vi "globalDevices.vi"() -> ()   [LabVIEW 2017]
panel:
  out "hamamatsuFrameReferences":refnum<data-value>[](array[refnum])
  out "ludlError":errorcluster
  in  "ludlPort":refnum<visa-resource-name>="COM1"
  out "daqVolumeFileError":errorcluster
  out "daqVolumeFileRefnum":refnum<file>
  in  "autofocusAidStage":u16(ring) items=["none", "focusKnob"]
  out "flashTask":refnum<k21>
  out "flashError":errorcluster
  in  "flashDigitalLine":tag="Dev1/port0/line2"
  in  "focusKnobSpeed":u8=255
  out "focusKnobError":errorcluster
  in  "focusKnobPort":refnum<visa-resource-name>="COM1"
  out "piezoUSBLastWrittenPos (um)":dbl
  out "piezoUSBError":i32
  out "piezoUSBHandle":i32
  out "csuShutterLastStatus":bool
  out "csuError":errorcluster
  in  "csuPort":refnum<visa-resource-name>="COM1"
  in  "galvoDY":dbl=0.08
  in  "galvoDX":dbl=0.08
  in  "galvoY0":dbl=0.05
  in  "galvoX0":dbl=-0.03
  out "hamamatsuSubtractBG":bool=TRUE
  out "daqFileError":errorcluster
  out "daqFileRefnum":refnum<file>
  in  "daqAOBufferSize":i32=8191
  in  "piezoReadVolTimingThresh":dbl
  out "piezoReadVolTimingError":errorcluster
  out "piezoReadVolTimingTask":refnum<k21>
  in  "piezoReadVolTimingChannel":tag="Dev1/ai1"
  in  "piezoWriteFunctionType":u16(ring) items=["triangle", "sine"]
  in  "galvoWriteMinVal":dbl=-10.0
  in  "galvoWriteMaxVal":dbl=10.0
  out "galvoYWriteError":errorcluster
  out "galvoXWriteError":errorcluster
  out "galvoYWriteTask":refnum<k21>
  out "galvoXWriteTask":refnum<k21>
  in  "galvoVoltsPerDegree":dbl=0.8
  in  "galvoYWriteChannel":tag="Dev2/ao0"
  in  "galvoXWriteChannel":tag="Dev2/ao1"
  in  "pharosClockRate":dbl=500000.0
  out "piezoWriteInitAtCenter":bool=TRUE
  out "piezoWriteInitRamp":dbl[](array[numeric])
  in  "piezoWriteSamplingRate":dbl=5000.0
  out "filterWheelInitialStatus":string
  out "filterWheelError":errorcluster
  in  "filterWheelPort":refnum<visa-resource-name>="COM1"
  in  "piezoWriteMaxVal":dbl=10.0
  out "hamamatsuStartTriggerMode":bool
  in  "piezoReadMinVal":dbl format="%0.2f"
  in  "piezoReadMaxVal":dbl=10.0 format="%0.2f"
  in  "piezoReadChannel":tag="Dev1/ai0"
  in  "hamamatsuFrameCounterTerminal":tag="/Dev1/PFI1"
  out "pharosError":errorcluster
  out "pharosTask":refnum<k21>
  in  "pharosDigitalLine":tag="Dev1/port0/line0"
  out "hamamatsuFrameCounterError":errorcluster
  out "hamamatsuFrameCounterTask":refnum<k21>
  in  "hamamatsuFrameCounterChannel":tag="Dev1/ctr0"
  in  "hamamatsuBufferSize":i32=200
  out "hamamatsuError":errorcluster {"code" format="%.0x"}
  out "hamamatsuBufferInfo":T1
  out "hamamatsuImageType":u32
  out "hamamatsuHandle":u32
  out "piezoWriteError":errorcluster
  out "piezoWriteTask":refnum<k21>
  in  "piezoWriteChannel":tag="Dev1/ao0"
  in  "piezo V/um":dbl=0.05
  out "piezoReadError":errorcluster
  out "piezoReadTask":refnum<k21>
  out "xboxError":errorcluster
  out "xboxID":refnum<k1>
  out "stageError":errorcluster
  out "stageIDs":cluster{"opaque pointer":u64, "id":i32}
  # "XBOX CONTROLLER"
  # "PIEZO"
  # "PHAROS"
  # "GALVO"
  # "STAGE (STANDA)"
  # "HAMAMATSU"
  # "FILTER WHEEL"
  # "Output (out from piezo)"
  # "Input (into piezo)"
  # "The galvo is mounted \"reversed\"\nwrt the labels on the motors. The\nmotor labelled \"X\" moves in Y and\nthe motor labelled \"Y\" moves in X.\n\nHere, I use the actual directions,\nnot the ones on the labels."
  # "CSU"
  # "FLASH"
  # "GENERAL DAQ"
  # "Volume timing"
  # "Frame counter"
  # "FOCUS KNOB"
  # "LUDL STAGE"
  # "USB connection"
  # "HARDWR CONFIG."
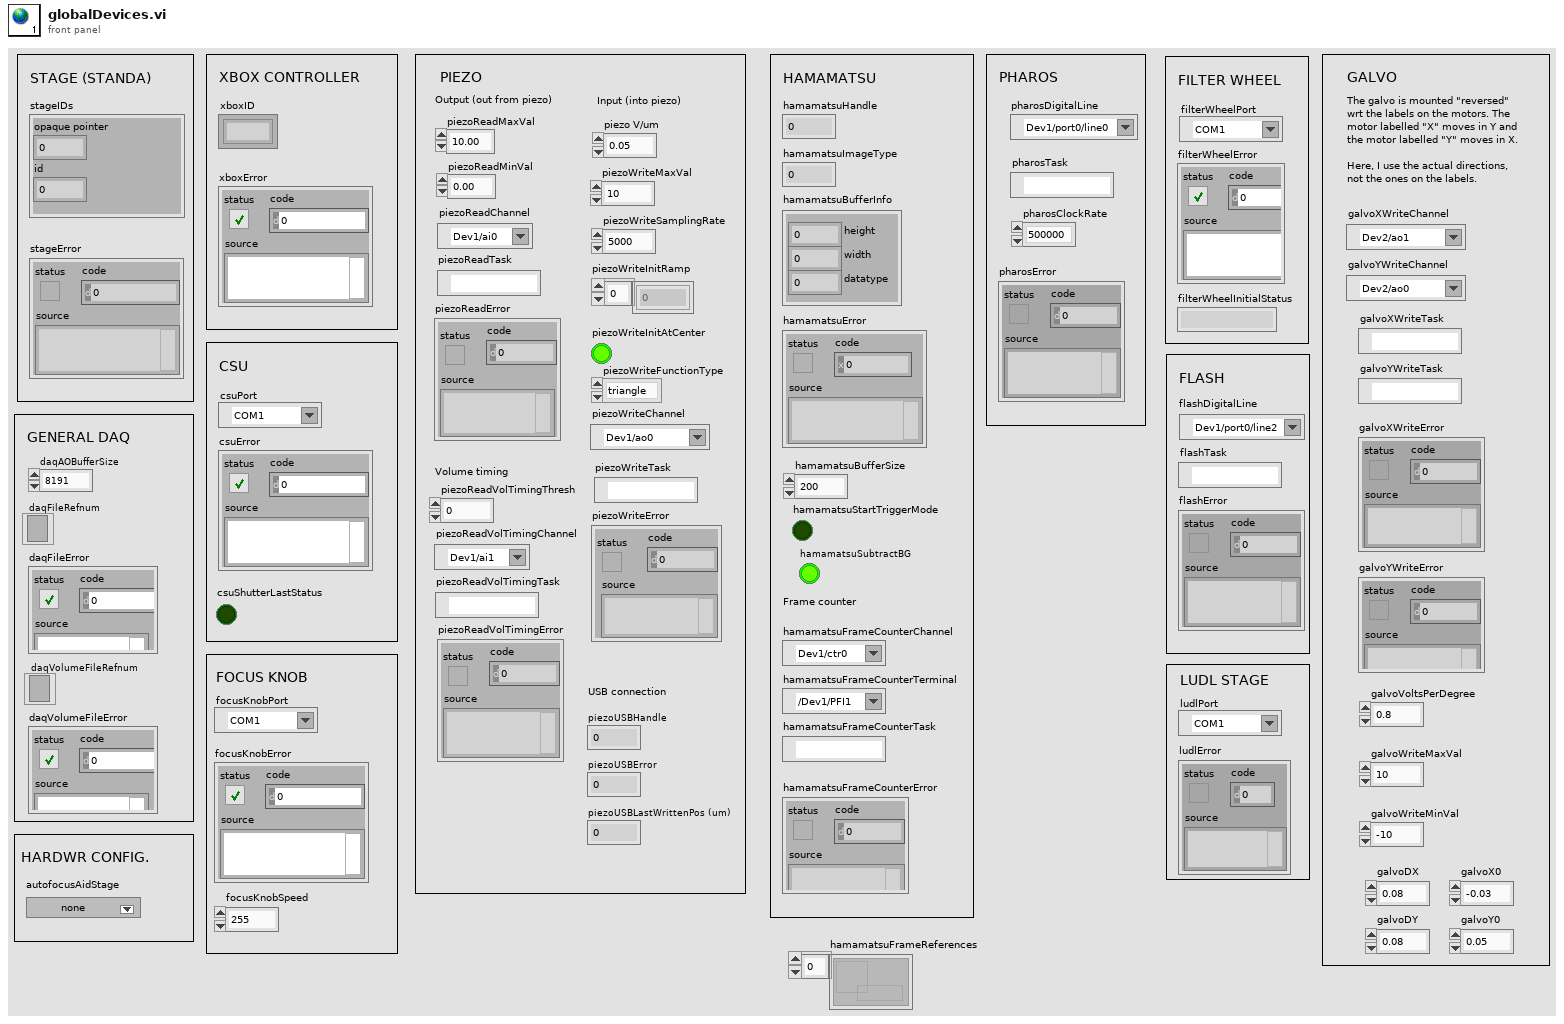
[diagram p1: front panel]
types:
  T1 = cluster{"height":i32, "width":i32, "datatype":i32}
diagram:
